vi "EXCEL OPEN.vi"(8 "error in (no error)":errorcluster, 10 "PATH IN":path=path "D:/LABVIEW TRIALS/USER.xlsx", 11 "Automation Refnum in":refnum<k7>) -> (0 "error out":errorcluster, 1 "PATH OUT":path, 2 "WORKBOOK OUT":refnum<k7>, 3 "Excel Application ref  out":refnum<k7>, 5 "WORKBOOKS REF OUT":refnum<k7>)   [LabVIEW 2021]
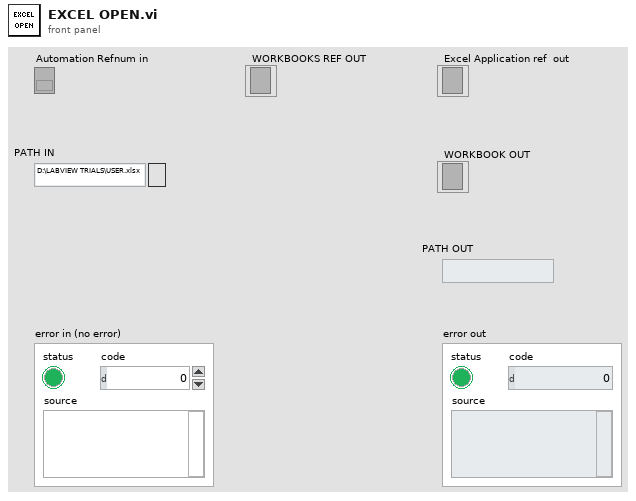
[diagram p1: front panel]
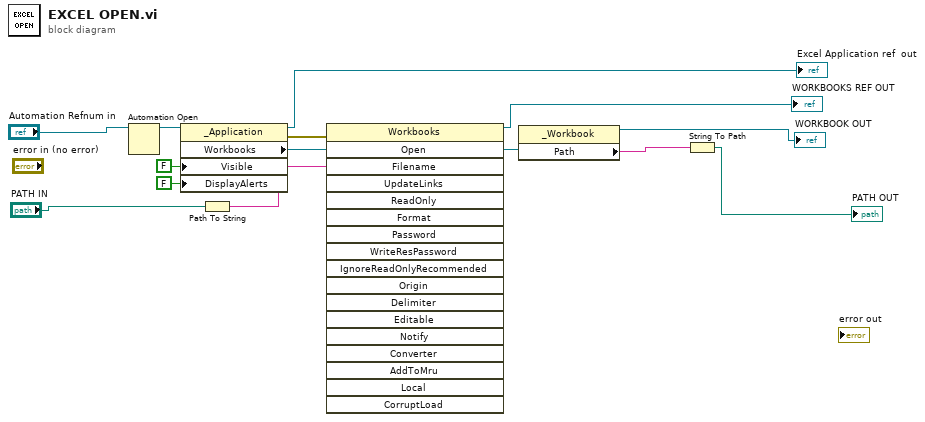
[diagram p0: block diagram]
diagram:
  n1 = Automation Open(Automation Refnum="Automation Refnum in") -> (Automation Refnum=w6:refnum<k7>)  [unwired: 3 in, 1 out]
  n2 = property class="_Application"(reference=w6, "Visible"=FALSE, "DisplayAlerts"=FALSE) -> (reference out=→"Excel Application ref  out":refnum<k7>, error out=w9:errorcluster, "Workbooks"=w10:refnum<k7>)  [unwired: 1 in]
  n3 = Path To String(path="PATH IN") -> (string=w11:string)
  n4 = invoke class="Workbooks" method="Open"(reference=w10, error in=w9, "Filename"=w11) -> (reference out=→"WORKBOOKS REF OUT":refnum<k7>, "Open"=w4:refnum<k7>)  [unwired: 15 in, 16 out]
  n5 = property class="_Workbook"(reference=w4) -> (reference out=→"WORKBOOK OUT":refnum<k7>, "Path"=w3:string)  [unwired: 1 in, 1 out]
  n6 = String To Path(string=w3) -> (path=→"PATH OUT":path)
